vi "UpdateFPReply.vi"(2 "success?":bool, 3 "Reply":string, 4 "Sent":string, 5 "method":string) -> ()   [LabVIEW 2010]
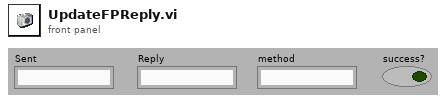
[diagram p1: front panel]
types:
  T1 = cluster{"Sent":string, "Reply":string, "method":string, "success?":bool, "element":string, "element":string}
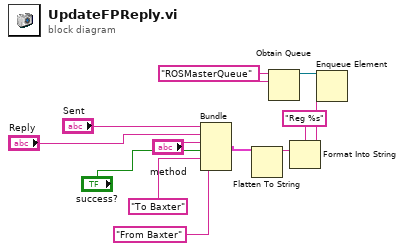
[diagram p0: block diagram]
diagram:
  w3 = "ROSMasterQueue" ("name (unnamed)")
  n1 = Bundle("Sent"="Sent", "Reply"="Reply", "method"="method", "success?"="success?", "element"="To Baxter", "element"="From Baxter") -> (w10:T1)  [unwired: 1 in]
  n2 = Flatten To String(anything=w10) -> (data string=w11:string)  [unwired: 3 in, 2 out]
  n3 = Obtain Queue(name (unnamed)=w3, element data type=w3) -> (queue out=w4:refnum<queue>)  [unwired: 3 in, 2 out]
  n4 = Format Into String(format string="Reg %s" ("element"), w11) -> (resulting string=w12:string)  [unwired: 2 in, 1 out]
  n5 = Enqueue Element(queue=w4, element=w12) -> ()  [unwired: 2 in, 3 out]
